vi "Mercury_GCS_Sample_Application_1.vi"() -> ()   [LabVIEW 2011]
doc: "This VI demonstrates how to define a Mercury (with GCS firmware) configuration with a connected axis. In this example the Mercury is connected through COM port 1 with baudrate 38400. The VI runs Mercury_GCS_Configuration_Setup.vi with these specified settings and reads the position of all axes. The diagram shows how to combine the driver VIs for these tasks.\n\nWarning: Before running this VI, modify Interface and RS232 settings (or add USB settings if Interface = USB was selected) to reflect your configuration. The predefined settings provided with the VI probably do not match your system."
panel:
  in  "stop":bool
  in  "error in":errorcluster
  out "Running":bool caption="Mercury_GCS_Configuration_Setup.vi is running"
  out "error out":errorcluster
  out "Position":dbl[](array[numeric]) format="%.6f"
  out "Conn. Axis":string[](array[string])
  out "Identification":string
  # "Simple Mercury GCS sample program (one system)"
  # "This VI demonstrates how to define a Mercury GCS configuration with a connected axis. In this example the Mercury is connected through COM port 1 \nwith baudrate 38400. The VI runs Mercury_GCS_Configuration_Setup.vi with these specified settings and reads the position of the axis. The diagram \nshows how to combine the driver VIs for these tasks. \n\nWarning: Before running this VI, modify \"Interface\", \"RS232 settings\" (or add USB settings if Interface = USB was selected) to reflect\n                 your configuration. The predefined settings provided with the VI probably do not match your system."
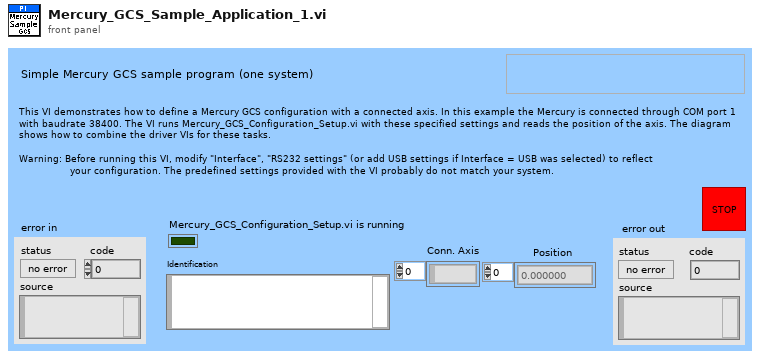
[diagram p1: front panel]
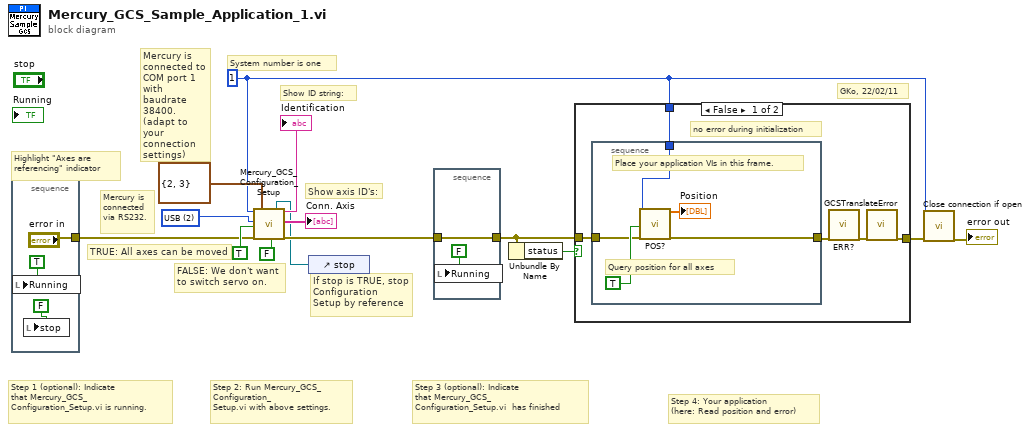
[diagram p0: block diagram]
diagram:
  w1 = u16 2 items=["RS232", "RS232 DaisyChain", "USB", "USB_DaisyChain"] ("Interface")
  w2 = 1 ("System no.")
  # "Mercury is\nconnected\nvia RS232."
  # "If stop is TRUE, stop \nConfiguration\nSetup by reference"
  # "Mercury is\nconnected to\nCOM port 1\nwith baudrate\n38400.\n(adapt to your\nconnection\nsettings)"
  # "GKo, 22/02/11"
  # "Step 4: Your application\n(here: Read position and error)"
  # "Step 3 (optional): Indicate\nthat Mercury_GCS_\nConfiguration_Setup.vi  has finished"
  # "Step 2: Run Mercury_GCS_\nConfiguration_\nSetup.vi with above settings."
  # "Step 1 (optional): Indicate\nthat Mercury_GCS_\nConfiguration_Setup.vi is running."
  # "Highlight \"Axes are\nreferencing\" indicator"
  # "Show axis ID's:"
  # "Show ID string:"
  # "FALSE: We don't want\nto switch servo on."
  # "TRUE: All axes can be moved"
  # "System number is one"
  n1 = stacked-sequence {
    tunnel: ["error in"] -> w10
    frame #0 {
      n2 = local write "Running"(TRUE ("Running")) -> ()
      n3 = local write "stop"(FALSE ("stop")) -> ()
    }
  }
  n4 = control-ref of="stop"() -> (w5:refnum<vi>)
  n5 = call "Mercury_GCS_Configuration_Setup.vi"("System no."=w2, "Interface"=w1, "All axes?"=TRUE, "error in"=w10, "RS232 settings"=cluster{"RS232 Portnumber":i32, "Baudrate":u16} {"RS232 Portnumber"=2, "Baudrate"=3}, "Switch servo on?"=FALSE ("Use dialog to define\nconnected stages?"), "Stop refnum"=w5) -> ("Identification"=→"Identification":string, "Conn. \nAxes"=→"Conn. Axis":string[], "error out"=w11:errorcluster)  [unwired: 6 in, 4 out]
  n6 = stacked-sequence {
    tunnel: w11 -> [w19]
    tunnel: [w19] -> w7
    frame #0 {
      n7 = local write "Running"(FALSE ("Running")) -> ()
    }
  }
  n8 = Unbundle By Name(w7) -> ("status"=w6:bool)
  n9 = case shown="False" w6 {
    tunnel: w2 -> [w24 _]
    tunnel: w7 -> [w23 w30]
    tunnel: [w20 w30] -> w4
    frame False {
      # "no error during initialization"
      n10 = stacked-sequence {
        tunnel: w24 -> [w29]
        tunnel: [w26] -> w21
        tunnel: w23 -> [w25]
        frame #0 {
          # "Place your application VIs in this frame."
          # "Query position for all axes"
          n11 = call "POS?.vi"("System no."=w29, "All axes?"=TRUE, "error in"=w25) -> ("Position"=→"Position":dbl[], "error out"=w26:errorcluster)  [unwired: 15 in]
        }
      }
      n12 = call "ERR?.vi"("error in"=w21) -> ("error out"=w22:errorcluster)  [unwired: 17 in, 1 out]
      n13 = call "GCSTranslateError.vi"("error in"=w22) -> ("error out"=w20:errorcluster)  [unwired: 16 in, 2 out]
    }
    frame True {
      # "error during initialization!"
    }
  }
  n14 = call "Close connection if open.vi"("System no."=w2, "error in"=w4) -> ("error out"=→"error out":errorcluster)  [unwired: 16 in, 1 out]
